vi "indent and spacing constant.vi"() -> (0 "indent and spacing":T1 {"At" format="%.2f"; "After" format="%.2f"; "Before" format="%.2f"; "By" format="%.2f"; "Right" format="%.2f"; "Left" format="%.2f"})   [LabVIEW 2010, in "NI_ReportGenerationToolkit.lvlib"]
doc: "Defines the indent and spacing attributes for a specified range within a Word document."
uses:
  <vilib>/addons/_office/NI_ReportGenerationToolkit.lvlib
panel:
  # "Indentation"
  # "Spacing"
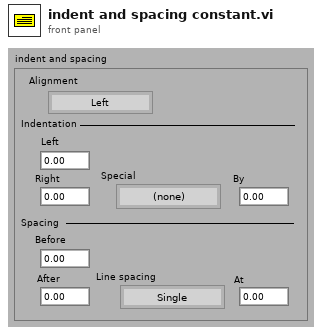
[diagram p1: front panel]
types:
  T1 = cluster{"Alignment":enum16{"Left", "Centered", "Right", "Justify"}, "Left":dbl, "Right":dbl, "Special":enum16{"(none)", "First line", "Hanging"}, "By":dbl, "Before":dbl, "After":dbl, "Line spacing":enum16{"Single", "1,5 lines", "Double", "At least", "Exactly", "Multiple"}, "At":dbl}
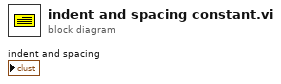
[diagram p0: block diagram]
diagram:
